vi "Main.vi"() -> ()   [LabVIEW 2017]
doc: "This Continuous Measurement sample project is based on the Queued Message Handler template.\n\nThe Event Handling Loop generates messages based on user interface actions.\n\nThe Message Handling Loop processes messages generated by the Event Handling Loop, or by other messages. There are also Acquisition and Logging message handling loop subVIs, and a chart updating loop."
uses:
  Settings/Settings.ctl
  Acquisition/Hardware Configuration.ctl
  Acquisition/Signal Type.ctl
  Logging/Logging Configuration.ctl
  controls/UI Data.ctl
  controls/UI State.ctl
  support/Message Queue/Enqueue Message (Single).vi
  support/Message Queue/Enqueue Message (Array).vi
  <vilib>/Utility/error.llb/Error Cluster From Error Code.vi
  <vilib>/ErrorRing/Error Ring.xnode
  Acquisition/Acquisition.lvlib
  Logging/Logging.lvlib
  Settings/Settings.lvlib
  support/User Event - Stop/User Event - Stop.lvlib
  support/Message Queue/Message Queue.lvlib
  Settings/Settings Dialog.vi
panel:
  in  "Zero run?":bool
  out "Max writing time to a file [min]":dbl
  out "Elapsed time":timestamp
  out "Test time zero run [s]":dbl
  out "Test time [s]":dbl
  in  "Start":bool
  in  "Stop":bool
  in  "Settings":bool
  out "Status":string
  in  "Exit":bool
  out "Log File Offsite Path":path
  out "Project code":string
  out "Offsite storage?":bool
  out "Log File Path":path
  out "Data":waveform(dbl)[](graph)
  # "Continuous Measurement Data Logger"
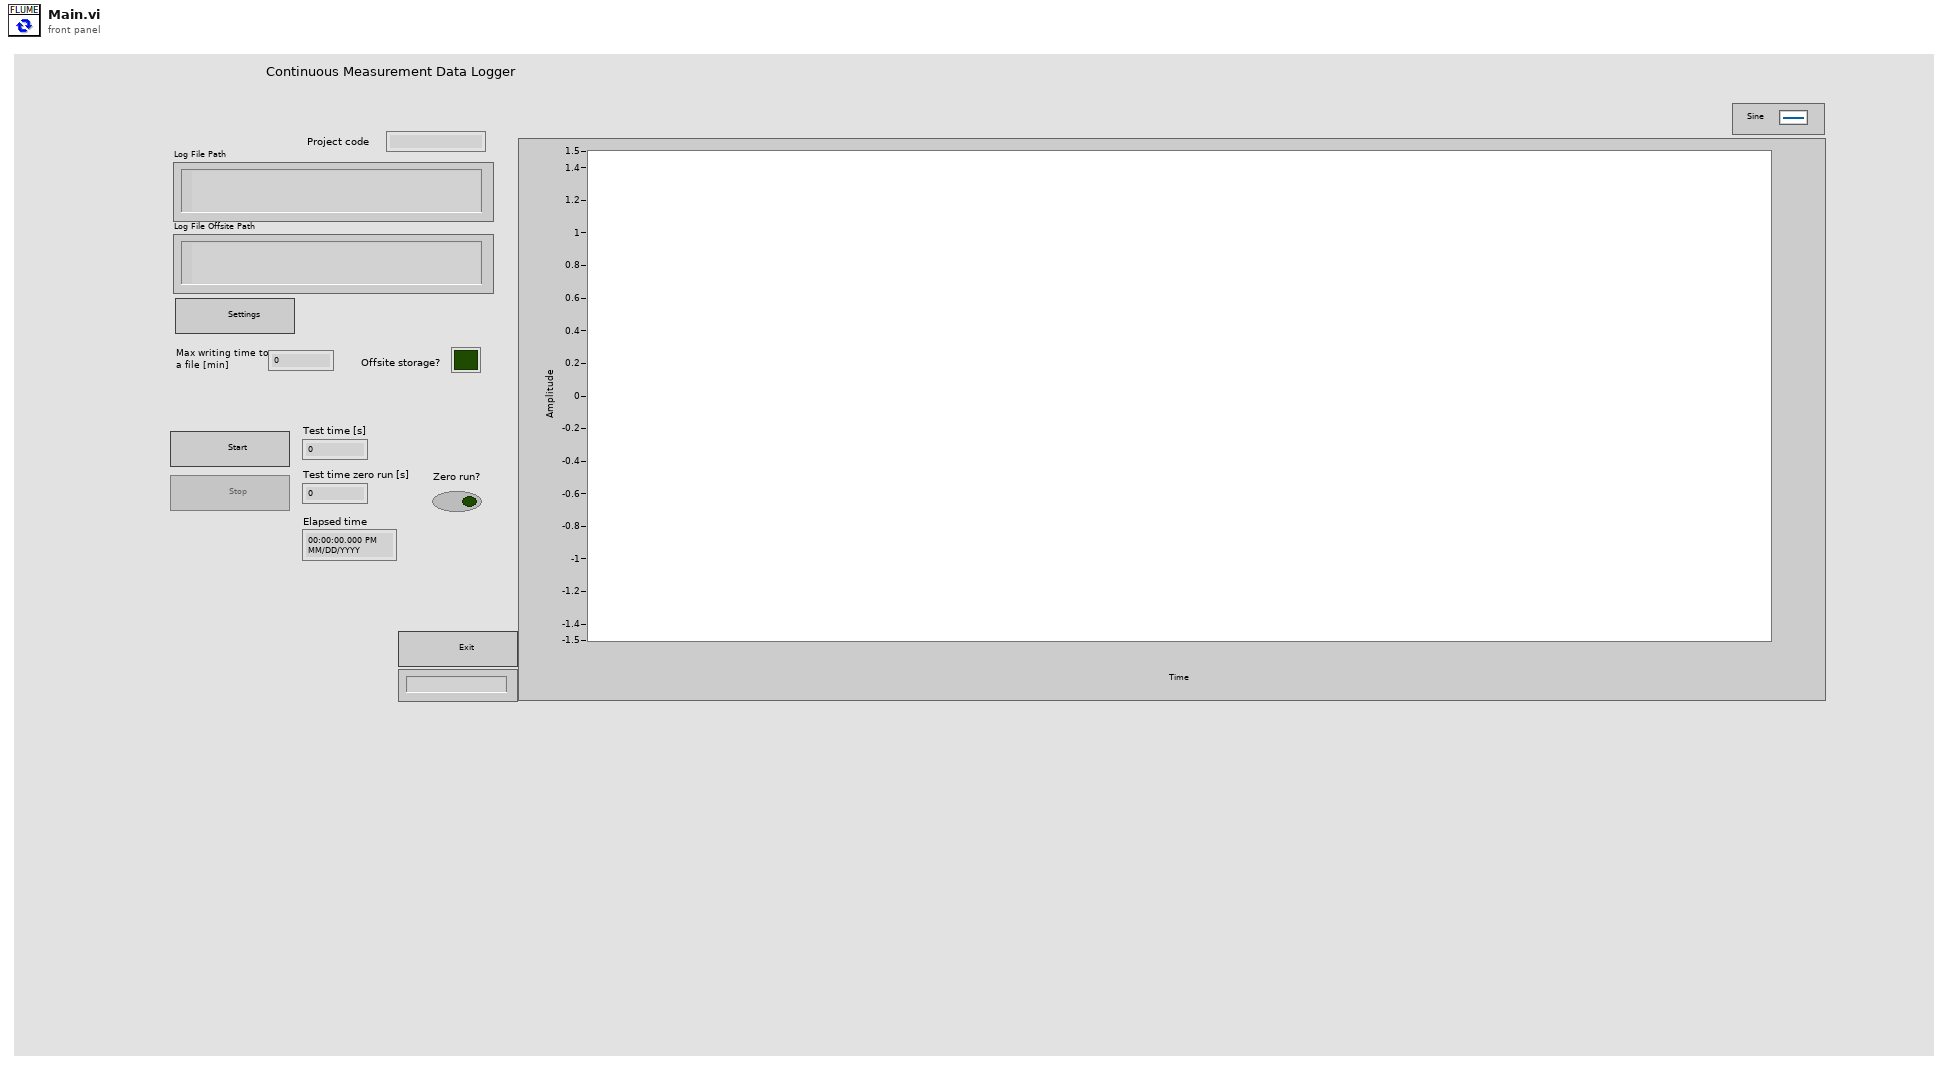
[diagram p1: front panel]
types:
  T1 = typedef "UI State.ctl" = enum16{"Idle", "Acquiring and Logging", "Waiting for Exit", "Waiting for Exit (Acq Stopped)", "Waiting for Exit (Log Stopped)", "Waiting for Stop", "Waiting for Stop (Acq Stopped)", "Waiting for Stop (Log Stopped)"}
  T2 = typedef "UI Data.ctl" = cluster{"Start Ref":refnum<vi>, "Stop Ref":refnum<vi>, "Settings Ref":refnum<vi>, "Exit Ref":refnum<vi>, "Status Ref":refnum<vi>, "Data Ref":refnum<vi>}
  T3 = typedef "Settings.lvlib/Settings.ctl" = cluster{"Hardware Configuration":T4, "Logging Configuration":T6, "Cluster":cluster{"Elapsed Time":dbl, "Test time [s]":dbl, "Test time zero run[s] ":dbl, "Zero run?":bool}}
  T4 = typedef "Acquisition.lvlib/Hardware Configuration.ctl" = cluster{"HW Refnum <Replace Me>":string, "Signal Type <Replace Me>":T5}
  T5 = typedef "Acquisition.lvlib/Signal Type.ctl" = enum16{"Sine Wave", "Square with Noise"}
  T6 = typedef "Logging.lvlib/Logging Configuration.ctl" = cluster{"Log File Base Path":path, "TDMS File Reference":refnum<k34>, "Log File Offsite Path":path, "Offsite storage?":bool, "Project code":string, "Max writing time to a file [min]":dbl}
  T7 = typedef "Message Queue.lvlib/All Message Queues.ctl" = cluster{"UI":refnum<queue>, "Acquisition":refnum<queue>, "Logging":refnum<queue>}
  T8 = cluster{"Elapsed Time":dbl, "Test time [s]":dbl, "Test time zero run[s] ":dbl, "Zero run?":bool}
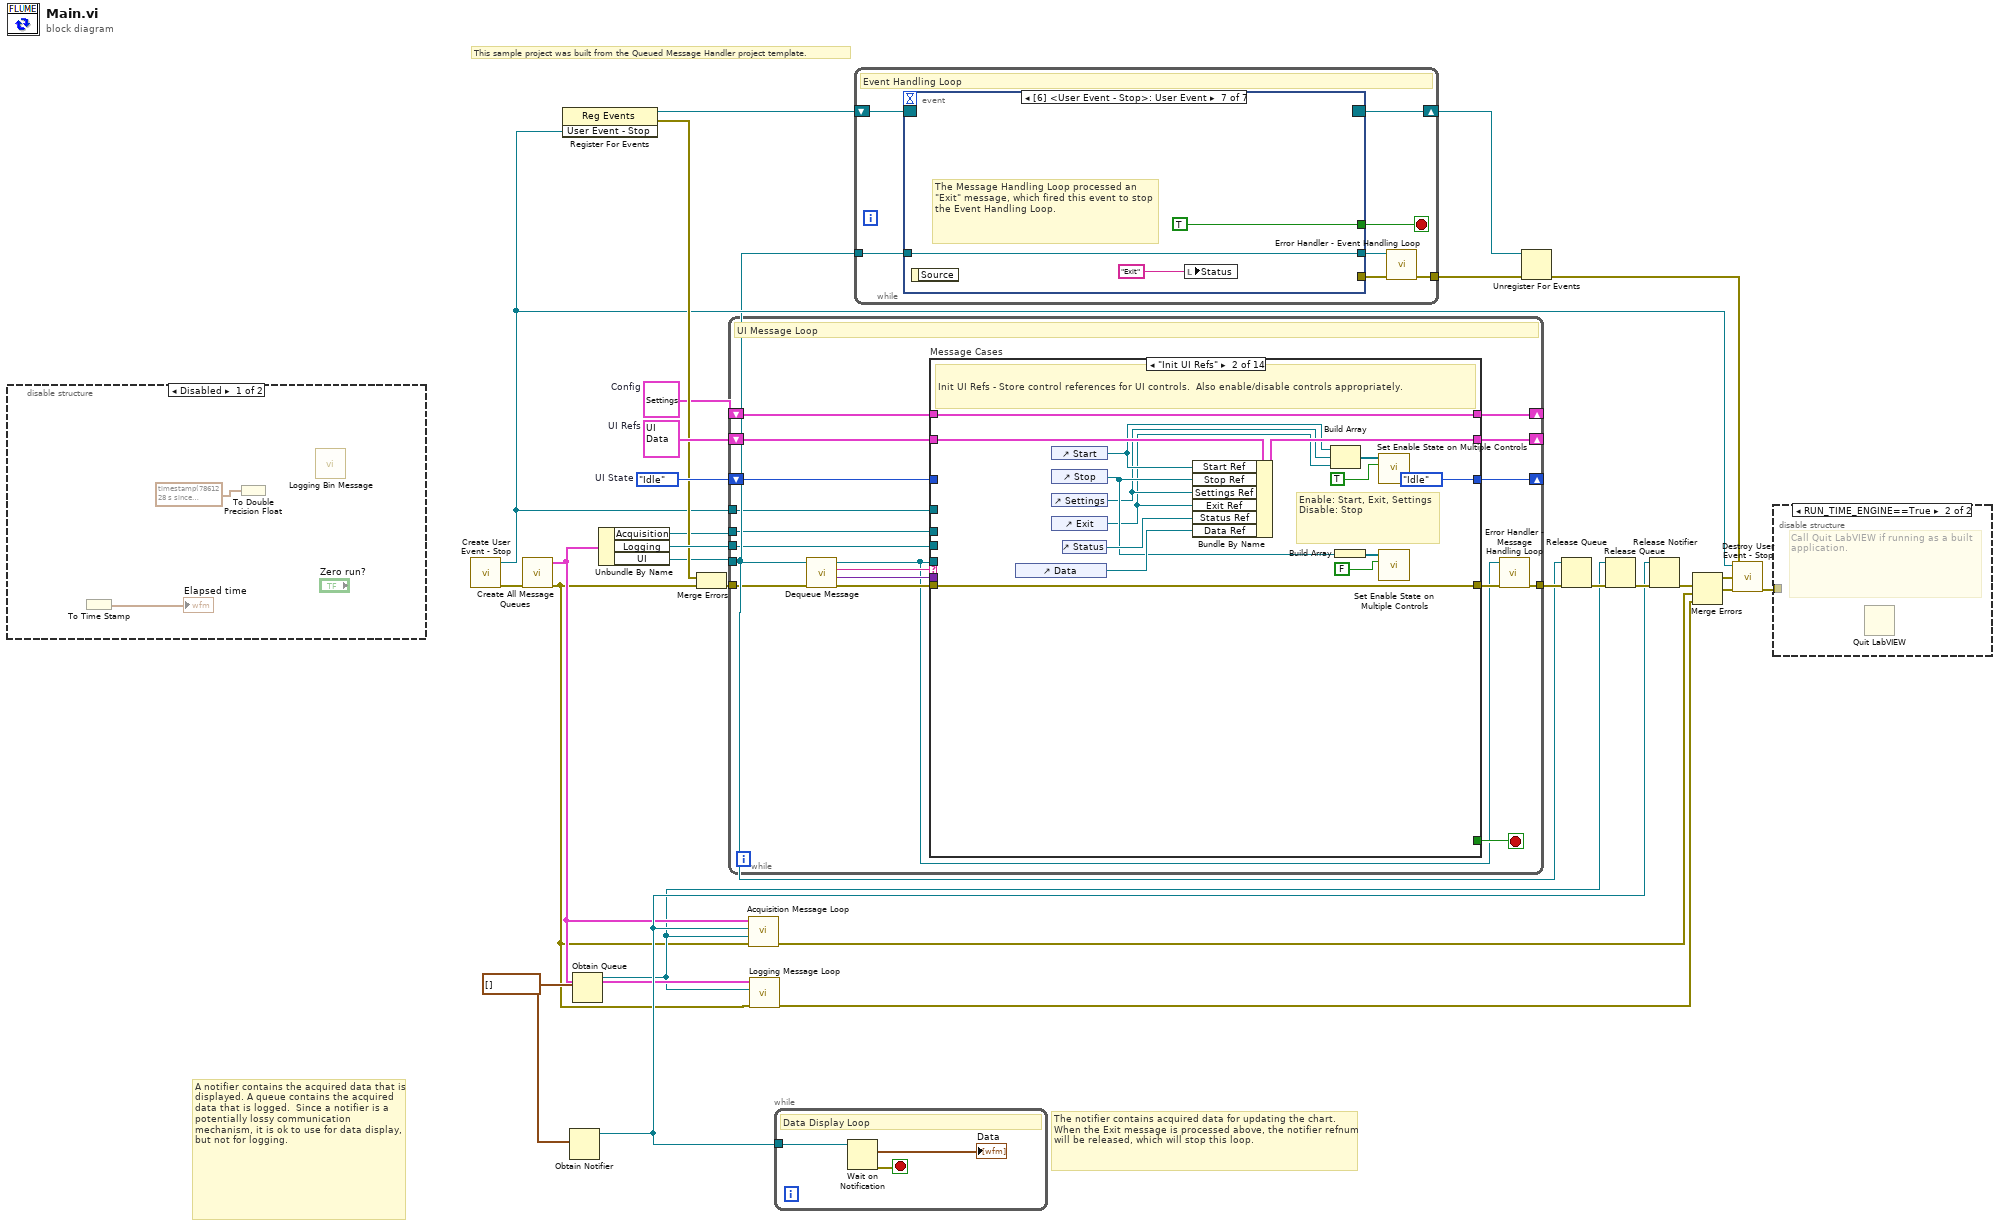
[diagram p0: block diagram]
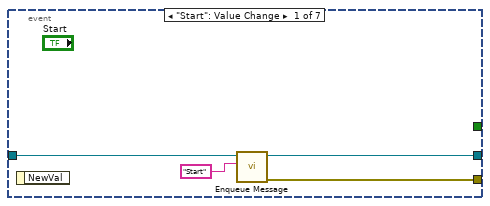
[diagram p4: hidden frame]
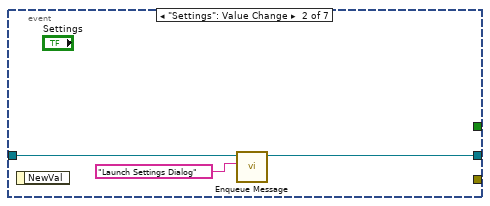
[diagram p5: hidden frame]
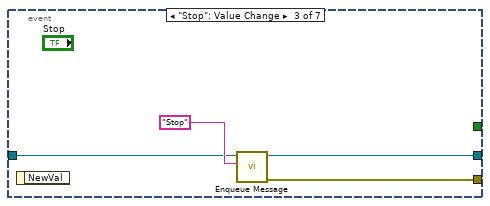
[diagram p6: hidden frame]
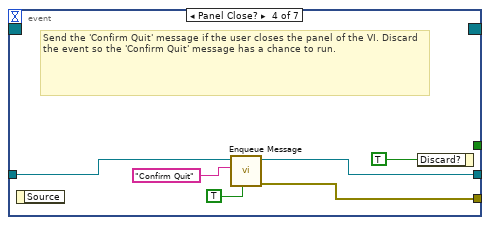
[diagram p7: hidden frame]
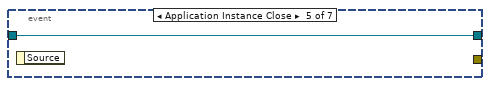
[diagram p8: hidden frame]
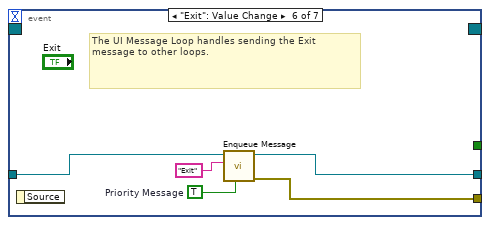
[diagram p9: hidden frame]
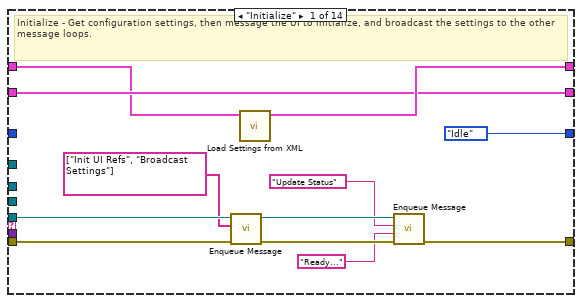
[diagram p10: hidden frame]
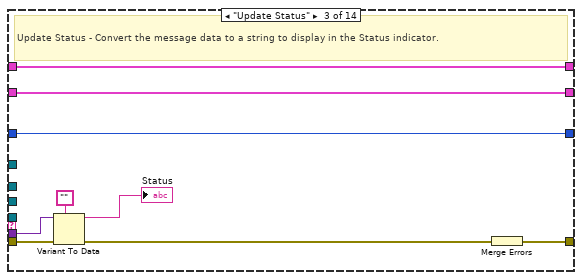
[diagram p11: hidden frame]
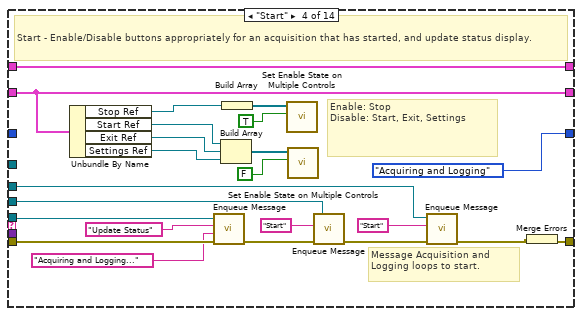
[diagram p12: hidden frame]
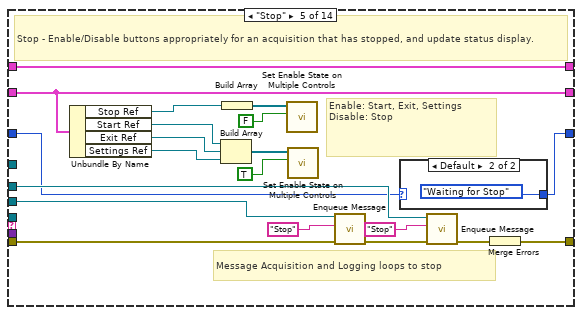
[diagram p13: hidden frame]
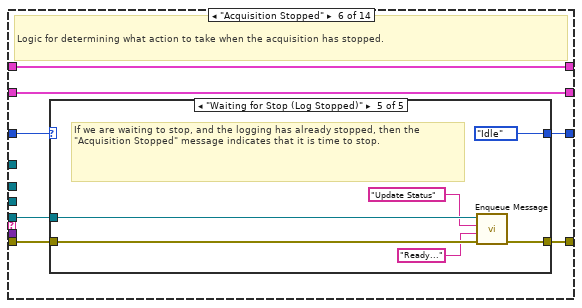
[diagram p15: hidden frame]
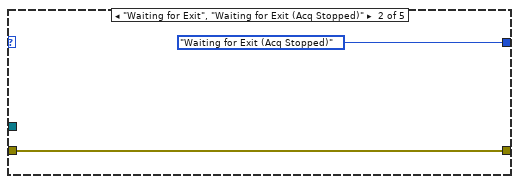
[diagram p17: hidden frame]
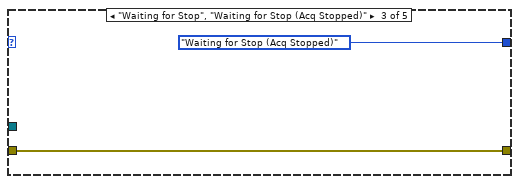
[diagram p18: hidden frame]
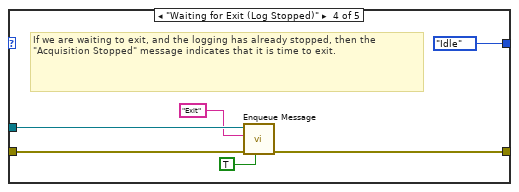
[diagram p19: hidden frame]
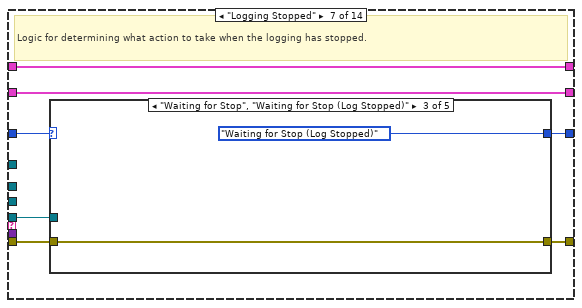
[diagram p20: hidden frame]
diagram:
  w19 = UI_State."Idle"  # UI State
  w4 = waveform(dbl)[] []
  w21 = T2 {"Start Ref"=refnum, "Stop Ref"=refnum, "Settings Ref"=refnum, "Exit Ref"=refnum, "Status Ref"=refnum, "Data Ref"=refnum}  # UI Refs
  w5 = T3 {"Hardware Configuration"={"HW Refnum <Replace Me>"="", "Signal Type <Replace Me>"=enum."Sine Wave"}, "Logging Configuration"={"Log File Base Path"=path "", "TDMS File Reference"=refnum, "Log File Offsite Path"=path "", "Offsite storage?"=FALSE, "Project code"="", "Max writing time to a file [min]"=0.0}, "Cluster"={"Elapsed Time"=0.0, "Test time [s]"=0.0, "Test time zero run[s] "=0.0, "Zero run?"=FALSE}}  # Config
  # "This sample project was built from the Queued Message Handler project template."
  # "A notifier contains the acquired data that is displayed. A queue contains the acquired data that is logged.  Since a notifier is a potentially lossy communication mechanism, it is ok to use for data display, but not for logging."
  # "The notifier contains acquired data for updating the chart. When the Exit message is processed above, the notifier refnum will be released, which will stop this loop."
  n1 = disable-structure shown="Disabled" {
    frame Disabled {
      n2 = To Time Stamp() -> (0:→"Elapsed time":timestamp)  [unwired: 1 in]
      n3 = To Double Precision Float(number=timestamp(7861228 s since 1904-01-01)) -> ()  [unwired: 1 out]
      n4 = call "Logging Bin Message.vi"() -> ()  [unwired: 11 in, 1 out]
    }
    frame Enabled {
    }
  }
  n5 = call "Create User Event - Stop.vi"() -> ("error out"=w24:errorcluster, "User Event - Stop"=w10:refnum<user-event>)  [unwired: 10 in]
  n6 = call "Create All Message Queues.vi"("error in (no error)"=w24) -> ("error out"=w1:errorcluster, "Message Queues out"=w3:T7)  [unwired: 9 in]
  n7 = register-events(w10) -> (reference out=w13:refnum<event-registration>, error out=w11:errorcluster)  [unwired: 2 in]
  n8 = Obtain Notifier(notification data type=w4) -> (notifier out=w6:refnum<notifier>)  [unwired: 3 in, 2 out]
  n9 = Obtain Queue(element data type=w4) -> (queue out=w2:refnum<queue>)  [unwired: 4 in, 2 out]
  n10 = Unbundle By Name(w3) -> ("Acquisition"=w8:refnum<queue>, "Logging"=w20:refnum<queue>, "UI"=w9:refnum<queue>)
  n11 = Merge Errors(w11, w1) -> (w12:errorcluster)
  n12 = while {
    tunnel: w9 -> [w32]
    tunnel: w10 -> [w46]
    shift-right: [w41] -> _
    shift-left: w5 -> [w40]
    shift-right: [w38] -> _
    shift-left: w21 -> [w39]
    tunnel: w8 -> [w37]
    tunnel: w20 -> [w31]
    shift-right: [w33] -> _
    shift-left: w19 -> [w34]
    tunnel: w12 -> [w45]
    tunnel: [w36] -> w27
    stop <- w47 stop-if-true
    # "UI Message Loop"
    n13 = call "Dequeue Message.vi"("error in (no error)"=w45, "Message Queue"=w32) -> ("error out"=w44:errorcluster, "Message Data"=w42:variant, "Message"=w43:string, "dup Message Queue"=w30:refnum<queue>)  [unwired: 6 in]
    n14 = case "Message Cases" shown="\"Init UI Refs\"" w43 {
      selector: w43 -> [_ _ _ _ _ _ _ _ _ _ _ _ _ w272]
      tunnel: w30 -> [w52 _ _ w85 _ w132 w157 _ w204 _ w226 _ _ _]
      tunnel: w44 -> [w51 w74 w82 w106 w125 w133 w158 w193 w206 w214 w225 w254 w270 _]
      tunnel: [w56 w74 w83 w87 w126 w130 w155 w198 w200 w217 w224 w263 w269 w271] -> w35
      tunnel: [_ _ _ _ _ _ _ _ _ _ _ TRUE _ _] -> w47
      tunnel: w42 -> [_ _ w81 _ _ _ _ _ _ w218 _ w252 _ _]
      tunnel: w46 -> [_ _ _ _ _ _ _ _ _ _ _ w264 _ _]
      tunnel: [w59 w60 w75 w84 w107 w129 w154 w196 w199 w213 w222 w250 w268 w275] -> w41
      tunnel: w40 -> [w48 w60 w75 w84 w107 w129 w154 w196 w207 w213 w222 w250 w268 w275]
      tunnel: w39 -> [w53 w73 w77 w103 w124 w135 w160 w191 w202 w221 w228 w262 w267 w274]
      tunnel: [w53 w70 w77 w103 w124 w135 w160 w191 w202 w221 w228 w262 w267 w274] -> w38
      tunnel: w37 -> [_ _ _ w86 w111 _ _ w190 _ _ _ w261 _ _]
      tunnel: w31 -> [_ _ _ w92 w114 _ _ w189 _ _ _ w260 _ _]
      tunnel: w34 -> [_ _ w76 _ w108 w134 w159 w188 w201 w216 w227 _ w266 w273]
      tunnel: [UI_State."Idle" ("UI State") UI_State."Idle" ("UI State") w76 UI_State."Acquiring and Logging" ("UI State") w109 w131 w156 w188 w201 w216 w223 UI_State."Idle" ("UI State") w266 w273] -> w33
      frame "Initialize" {
        # "Initialize - Get configuration settings, then message the UI to initialize, and broadcast the settings to the other message loops."
        n15 = call-poly "Enqueue Message.vi"("error in (no error)"=w51, "Message Array"=string[] ["Init UI Refs", "Broadcast Settings"], "Message Queue"=w52) -> ("error out"=w58:errorcluster, "dup Message Queue"=w57:refnum<queue>)  [unwired: 7 in]
        n16 = call "Load Settings from XML.vi"("Settings in"=w48) -> ("Settings out"=w59:T3)  [unwired: 9 in, 1 out]
        n17 = call-poly "Enqueue Message.vi"("error in (no error)"=w58, "Message Data"="Ready..." ("Ready..."), "Message"="Update Status", "Message Queue"=w57) -> ("error out"=w56:errorcluster)  [unwired: 6 in, 1 out]
      }
      frame "Init UI Refs" {
        # "Enable: Start, Exit, Settings\nDisable: Stop"
        # "Init UI Refs - Store control references for UI controls.  Also enable/disable controls appropriately."
        n18 = control-ref of="Data"() -> (w71:refnum<vi>)
        n19 = control-ref of="Start"() -> (w64:refnum<vi>)
        n20 = control-ref of="Stop"() -> (w65:refnum<vi>)
        n21 = control-ref of="Settings"() -> (w63:refnum<vi>)
        n22 = control-ref of="Exit"() -> (w62:refnum<vi>)
        n23 = control-ref of="Status"() -> (w72:refnum<vi>)
        n24 = Bundle By Name(cluster=w73, "Start Ref"=w64, "Stop Ref"=w65, "Settings Ref"=w63, "Exit Ref"=w62, "Status Ref"=w72, "Data Ref"=w71) -> (w70:T2)
        n25 = Build Array(w64, w63, w62) -> (w68:refnum<vi>[])
        n26 = Build Array(w65) -> (w67:refnum<vi>[])
        n27 = call "Set Enable State on Multiple Controls.vi"("Enable?"=TRUE, "Controls"=w68) -> ()  [unwired: 10 in]
        n28 = call "Set Enable State on Multiple Controls.vi"("Enable?"=FALSE, "Controls"=w67) -> ()  [unwired: 10 in]
      }
      frame "Update Status" {
        # "Update Status - Convert the message data to a string to display in the Status indicator."
        n29 = Variant To Data(error in=w82, type="", Variant=w81) -> (data=→"Status":string, error out=w79:errorcluster)
        n30 = Merge Errors(w79) -> (w83:errorcluster)
      }
      frame "Start" {
        # "Message Acquisition and Logging loops to start."
        # "Enable: Stop\nDisable: Start, Exit, Settings"
        # "Start - Enable/Disable buttons appropriately for an acquisition that has started, and update status display."
        n31 = Unbundle By Name(w103) -> ("Stop Ref"=w98:refnum<vi>, "Start Ref"=w97:refnum<vi>, "Exit Ref"=w96:refnum<vi>, "Settings Ref"=w95:refnum<vi>)
        n32 = call-poly "Enqueue Message.vi"("error in (no error)"=w106, "Message Data"="Acquiring and Logging..." ("Acquiring and Logging..."), "Message"="Update Status", "Message Queue"=w85) -> ("error out"=w94:errorcluster)  [unwired: 6 in, 1 out]
        n33 = Build Array(w97, w96, w95) -> (w101:refnum<vi>[])
        n34 = Build Array(w98) -> (w100:refnum<vi>[])
        n35 = call "Set Enable State on Multiple Controls.vi"("Enable?"=TRUE, "Controls"=w100) -> ()  [unwired: 10 in]
        n36 = call "Set Enable State on Multiple Controls.vi"("Enable?"=FALSE, "Controls"=w101) -> ()  [unwired: 10 in]
        n37 = call-poly "Enqueue Message.vi"("error in (no error)"=w94, "Message"="Start", "Message Queue"=w92) -> ("error out"=w89:errorcluster)  [unwired: 7 in, 1 out]
        n38 = call-poly "Enqueue Message.vi"("error in (no error)"=w89, "Message"="Start", "Message Queue"=w86) -> ("error out"=w88:errorcluster)  [unwired: 7 in, 1 out]
        n39 = Merge Errors(w88) -> (w87:errorcluster)
      }
      frame "Stop" {
        # "Message Acquisition and Logging loops to stop"
        # "Enable: Start, Exit, Settings\nDisable: Stop"
        # "Stop - Enable/Disable buttons appropriately for an acquisition that has stopped, and update status display."
        n40 = Unbundle By Name(w124) -> ("Stop Ref"=w119:refnum<vi>, "Start Ref"=w118:refnum<vi>, "Exit Ref"=w117:refnum<vi>, "Settings Ref"=w116:refnum<vi>)
        n41 = Build Array(w118, w117, w116) -> (w122:refnum<vi>[])
        n42 = Build Array(w119) -> (w121:refnum<vi>[])
        n43 = call "Set Enable State on Multiple Controls.vi"("Enable?"=FALSE, "Controls"=w121) -> ()  [unwired: 10 in]
        n44 = call "Set Enable State on Multiple Controls.vi"("Enable?"=TRUE, "Controls"=w122) -> ()  [unwired: 10 in]
        n45 = call-poly "Enqueue Message.vi"("error in (no error)"=w125, "Message"="Stop", "Message Queue"=w114) -> ("error out"=w113:errorcluster)  [unwired: 7 in, 1 out]
        n46 = case shown="Default" w108 {
          selector: w108 -> [w127 _]
          tunnel: [w127 UI_State."Waiting for Stop" ("UI State")] -> w109
          frame "Waiting for Exit" {
          }
          frame Default {
          }
        }
        n47 = call-poly "Enqueue Message.vi"("error in (no error)"=w113, "Message"="Stop", "Message Queue"=w111) -> ("error out"=w112:errorcluster)  [unwired: 7 in, 1 out]
        n48 = Merge Errors(w112) -> (w126:errorcluster)
      }
      frame "Acquisition Stopped" {
        # "Logic for determining what action to take when the acquisition has stopped."
        n49 = case shown="\"Waiting for Stop (Log Stopped)\"" w134 {
          selector: w134 -> [w137 _ _ _ _]
          tunnel: w133 -> [w136 w139 w141 w147 w153]
          tunnel: w132 -> [_ _ _ w145 w150]
          tunnel: [w137 UI_State."Waiting for Exit (Acq Stopped)" ("UI State") UI_State."Waiting for Stop (Acq Stopped)" ("UI State") UI_State."Idle" ("UI State") UI_State."Idle" ("UI State")] -> w131
          tunnel: [w136 w139 w141 w146 w151] -> w130
          frame Default {
          }
          frame "Waiting for Exit", "Waiting for Exit (Acq Stopped)" {
          }
          frame "Waiting for Stop", "Waiting for Stop (Acq Stopped)" {
          }
          frame "Waiting for Exit (Log Stopped)" {
            # "If we are waiting to exit, and the logging has already stopped, then the \"Acquisition Stopped\" message indicates that it is time to exit."
            n50 = call-poly "Enqueue Message.vi"("Priority Message? (F)"=TRUE, "error in (no error)"=w147, "Message"="Exit", "Message Queue"=w145) -> ("error out"=w146:errorcluster)  [unwired: 6 in, 1 out]
          }
          frame "Waiting for Stop (Log Stopped)" {
            # "If we are waiting to stop, and the logging has already stopped, then the \"Acquisition Stopped\" message indicates that it is time to stop."
            n51 = call-poly "Enqueue Message.vi"("error in (no error)"=w153, "Message Data"="Ready..." ("Ready..."), "Message"="Update Status", "Message Queue"=w150) -> ("error out"=w151:errorcluster)  [unwired: 6 in, 1 out]
          }
        }
      }
      frame "Logging Stopped" {
        # "Logic for determining what action to take when the logging has stopped."
        n52 = case shown="\"Waiting for Stop\", \"Waiting for Stop (Log Stopped)\"" w159 {
          selector: w159 -> [w162 _ _ _ _]
          tunnel: w158 -> [w161 w164 w166 w172 w175]
          tunnel: w157 -> [_ _ _ w170 w174]
          tunnel: [w162 UI_State."Waiting for Exit (Log Stopped)" ("UI State") UI_State."Waiting for Stop (Log Stopped)" ("UI State") UI_State."Idle" ("UI State") UI_State."Idle" ("UI State")] -> w156
          tunnel: [w161 w164 w166 w171 w173] -> w155
          frame Default {
          }
          frame "Waiting for Exit", "Waiting for Exit (Log Stopped)" {
          }
          frame "Waiting for Stop", "Waiting for Stop (Log Stopped)" {
          }
          frame "Waiting for Exit (Acq Stopped)" {
            # "If we are waiting to exit, and the acquisition has already stopped, then the \"Logging Stopped\" message indicates that it is time to exit."
            n53 = call-poly "Enqueue Message.vi"("Priority Message? (F)"=TRUE, "error in (no error)"=w172, "Message"="Exit", "Message Queue"=w170) -> ("error out"=w171:errorcluster)  [unwired: 6 in, 1 out]
          }
          frame "Waiting for Stop (Acq Stopped)" {
            # "If we are waiting to stop, and the acquisition has already stopped, then the \"Logging Stopped\" message indicates that it is time to stop."
            n54 = call-poly "Enqueue Message.vi"("error in (no error)"=w175, "Message Data"="Ready..." ("Ready..."), "Message"="Update Status", "Message Queue"=w174) -> ("error out"=w173:errorcluster)  [unwired: 6 in, 1 out]
          }
        }
      }
      frame "Broadcast settings" {
        w192 = "Update Settings" ("Message")
        # "Broadcast settings - Send the 'Update Settings' message to the Logging and Acquisition message loops."
        n55 = Unbundle By Name(w196) -> ("Hardware Configuration"=w195:T4, "Logging Configuration"=w185:T6, "Cluster"=w183:T8)
        n56 = Unbundle By Name(w183) -> ("Test time [s]"=→"Test time [s]":dbl, "Test time zero run[s]"=→"Test time zero run [s]":dbl)
        n57 = Unbundle By Name(w185) -> ("Log File Base Path"=→"Log File Path":path, "Log File Offsite Path"=→"Log File Offsite Path":path, "Offsite storage?"=→"Offsite storage?":bool, "Project code"=→"Project code":string, "Max writing time to a file [min]"=→"Max writing time to a file [min]":dbl)
        n58 = call-poly "Enqueue Message.vi"("Message Data"=w195, "Message"=w192, "Message Queue"=w190) -> ("error out"=w197:errorcluster)  [unwired: 7 in, 1 out]
        n59 = call-poly "Enqueue Message.vi"("error in (no error)"=w197, "Message Data"=w185, "Message"=w192, "Message Queue"=w189) -> ("error out"=w194:errorcluster)  [unwired: 6 in, 1 out]
        n60 = Merge Errors(w194, w193) -> (w198:errorcluster)
      }
      frame "Launch Settings Dialog" {
        # "Launch Settings Dialog - Launch the Settings Dialog when the user clicks the 'Settings' button."
        n61 = call-by-ref "?"("error in (no error)"=w206, "Settings in"=w207) -> ("error out"=w203:errorcluster, "Cancelled?"=w205:bool, "Settings out"=w199:T3)  [unwired: 8 in, 3 out]
        n62 = case shown="False" w205 {
          tunnel: w204 -> [w211 _]
          tunnel: w203 -> [w210 w212]
          tunnel: [w209 w212] -> w200
          frame False {
            n63 = call-poly "Enqueue Message.vi"("error in (no error)"=w210, "Message"="Broadcast Settings", "Message Queue"=w211) -> ("error out"=w209:errorcluster)  [unwired: 7 in, 1 out]
          }
          frame True {
          }
        }
      }
      frame "Error" {
        # "Error - Display an error dialog. This message is sent by the \"Error Handler\" VIs at the end of other loops in this application."
        n64 = Variant To Data(error in=w214, type=errorcluster {"status"=FALSE, "code"=0, "source"=""} ("error constant"), Variant=w218) -> (data=w215:errorcluster, error out=w219:errorcluster)
        n65 = call <vilib>:"Simple Error Handler.vi"("error in (no error)"=w215) -> ()  [unwired: 4 in, 5 out]
        n66 = Merge Errors(w219) -> (w217:errorcluster)
      }
      frame "Confirm Quit" {
        # "Confirm Quit - Message that can confirm whether or not the user wants to exit the application."
        n67 = case shown="\"Acquiring and Logging\"" w227 {
          tunnel: w226 -> [w234 w238]
          tunnel: w225 -> [w233 w237]
          tunnel: [w232 w236] -> w224
          tunnel: [UI_State."Idle" ("UI State") w235] -> w223
          frame Default {
            # "If 'Confirm Quit' comes in while the system is idle, there is no need for a confirmation message."
            n68 = call-poly "Enqueue Message.vi"("Priority Message? (F)"=TRUE, "error in (no error)"=w233, "Message"="Exit", "Message Queue"=w234) -> ("error out"=w232:errorcluster)  [unwired: 6 in, 1 out]
          }
          frame "Acquiring and Logging" {
            n69 = Two Button Dialog(message="Are you sure you want to quit while the acquisition is running?" ("Confirm Quit Message"), 1:"No" ("No"), 2:"Yes" ("Yes")) -> (T button?=w239:bool)
            n70 = case shown="True" w239 {
              tunnel: w238 -> [_ w248]
              tunnel: w237 -> [w244 w249]
              tunnel: [w244 w247] -> w236
              tunnel: [UI_State."Acquiring and Logging" ("UI State") UI_State."Waiting for Exit" ("UI State")] -> w235
              frame False {
                # "User did not want to quit."
              }
              frame True {
                n71 = call-poly "Enqueue Message.vi"("error in (no error)"=w249, "Message"="Stop", "Message Queue"=w248) -> ("error out"=w247:errorcluster)  [unwired: 7 in, 1 out]
              }
            }
          }
        }
      }
      frame "Exit" {
        w256 = TRUE ("Priority Message? (F)")
        w257 = "Exit" ("Message")
        # "Popup an error dialog if 'Exit' was called as a result of an error."
        # "Stop the VI"
        # "Exit - Send Exit messages to the Acquisition and Logging loops, and fire the user event to stop the Event Handling Loop."
        n72 = Variant To Data(type=errorcluster {"status"=FALSE, "code"=0, "source"=""} ("error constant"), Variant=w252) -> (data=w251:errorcluster)  [unwired: 1 in, 1 out]
        n73 = call <vilib>:"Simple Error Handler.vi"("error in (no error)"=w251) -> ()  [unwired: 4 in, 5 out]
        n74 = call-poly "Enqueue Message.vi"("Priority Message? (F)"=w256, "error in (no error)"=w254, "Message"=w257, "Message Queue"=w261) -> ("error out"=w258:errorcluster)  [unwired: 6 in, 1 out]
        n75 = call-poly "Enqueue Message.vi"("Priority Message? (F)"=w256, "error in (no error)"=w258, "Message"=w257, "Message Queue"=w260) -> ("error out"=w255:errorcluster)  [unwired: 6 in, 1 out]
        n76 = call "Fire User Event - Stop.vi"("error in (no error)"=w255, "User Event - Stop"=w264) -> ("error out"=w263:errorcluster)  [unwired: 9 in]
      }
      frame "---Copy This Frame---" {
        (unwired) FALSE ("Time has Elapsed")
        # "Duplicate this frame when creating new messages.  Change this comment in the duplicated frame to describe this message."
        n77 = Merge Errors(w270) -> (w269:errorcluster)
      }
      frame Default {
        # "'Default' case only runs if there is a message that isn't defined in any of the other cases.  Output a programming error."
        n78 = xnode "Error Ring"("parameter 0"=w272) -> ("error out"=w271:errorcluster)
      }
    }
    n79 = call "Error Handler - Message Handling Loop.vi"("error in (no error)"=w35, "Message Queue"=w30) -> ("dup error in"=w36:errorcluster)  [unwired: 8 in, 1 out]
  }
  n80 = call "Acquisition Message Loop.vi"("error in (no error)"=w1, "Data Queue"=w2, "Data Notifier"=w6, "Message Queues"=w3) -> ("error out"=w25:errorcluster)  [unwired: 7 in]
  n81 = call "Logging Message Loop.vi"("error in (no error)"=w1, "Data Queue"=w2, "Message Queues"=w3) -> ("error out"=w23:errorcluster)  [unwired: 8 in]
  n82 = while "Data Display Loop" {
    tunnel: w6 -> [w285]
    stop <- w284 stop-if-true
    # "Data Display Loop"
    n83 = Wait on Notification(notifier=w285) -> (notification=→"Data":waveform(dbl)[], error out=w284:errorcluster)  [unwired: 3 in, 2 out]
  }
  n84 = while {
    tunnel: w9 -> [w291]
    tunnel: [w288] -> w26
    shift-right: [w290] -> w22
    shift-left: w13 -> [w292]
    stop <- w289 stop-if-true
    # "Event Handling Loop"
    n85 = event shown="[6] <User Event - Stop>: User Event" {
      selector: w292 -> [_ _ _ _ _ _ _]
      dyn-events: [_ _ _ _ _ _ _] -> w290
      timeout: _ -> [_ _ _ _ _ _ _]
      tunnel: [_ _ _ _ _ _ TRUE ("Discard?")] -> w289
      tunnel: w291 -> [w296 w298 w302 w307 w310 w312 w316]
      tunnel: [w294 _ w301 w305 _ w315 _] -> w287
      tunnel: [w293 w297 w300 w306 w310 w311 w316] -> w286
      event "Start": Value Change {
        n86 = event-data() -> ()  [unwired: 1 in, 1 out]
        n87 = call-poly "Enqueue Message.vi"("Message"="Start", "Message Queue"=w296) -> ("error out"=w294:errorcluster, "dup Message Queue"=w293:refnum<queue>)  [unwired: 8 in]
      }
      event "Settings": Value Change {
        n88 = event-data() -> ()  [unwired: 1 in, 1 out]
        n89 = call-poly "Enqueue Message.vi"("Message"="Launch Settings Dialog", "Message Queue"=w298) -> ("dup Message Queue"=w297:refnum<queue>)  [unwired: 8 in, 1 out]
      }
      event "Stop": Value Change {
        n90 = event-data() -> ()  [unwired: 1 in, 1 out]
        n91 = call-poly "Enqueue Message.vi"("Message"="Stop", "Message Queue"=w302) -> ("error out"=w301:errorcluster, "dup Message Queue"=w300:refnum<queue>)  [unwired: 8 in]
      }
      event Panel Close? {
        # "Send the 'Confirm Quit' message if the user closes the panel of the VI. Discard the event so the 'Confirm Quit' message has a chance to run."
        n92 = event-data() -> ()  [unwired: 1 in, 1 out]
        n93 = call-poly "Enqueue Message.vi"("Priority Message? (F)"=TRUE, "Message"="Confirm Quit", "Message Queue"=w307) -> ("error out"=w305:errorcluster, "dup Message Queue"=w306:refnum<queue>)  [unwired: 7 in]
        n94 = event-data("Discard?"=TRUE) -> ()  [unwired: 1 in, 1 out]
      }
      event Application Instance Close {
        n95 = event-data() -> ()  [unwired: 1 in, 1 out]
      }
      event "Exit": Value Change {
        w313 = TRUE  # Priority Message
        # "The UI Message Loop handles sending the Exit message to other loops."
        n96 = event-data() -> ()  [unwired: 1 in, 1 out]
        n97 = call-poly "Enqueue Message.vi"("Priority Message? (F)"=w313, "Message"="Exit", "Message Queue"=w312) -> ("error out"=w315:errorcluster, "dup Message Queue"=w311:refnum<queue>)  [unwired: 7 in]
      }
      event User Event {
        # "The Message Handling Loop processed an \"Exit\" message, which fired this event to stop the Event Handling Loop."
        n98 = event-data() -> ()  [unwired: 1 in, 1 out]
        n99 = local write "Status"("Exit" ("Exit String")) -> ()
      }
    }
    n100 = call "Error Handler - Event Handling Loop.vi"("error in (no error)"=w287, "Message Queue"=w286) -> ("dup error in"=w288:errorcluster)  [unwired: 8 in, 1 out]
  }
  n101 = Unregister For Events(event registration refnum=w22, error in=w26) -> (error out=w7:errorcluster)
  n102 = Release Queue(queue=w9, error in (no error)=w27) -> (error out=w16:errorcluster)  [unwired: 1 in, 2 out]
  n103 = Release Queue(queue=w2, error in (no error)=w16) -> (error out=w15:errorcluster)  [unwired: 1 in, 2 out]
  n104 = Release Notifier(notifier=w6, error in (no error)=w15) -> (error out=w14:errorcluster)  [unwired: 1 in, 2 out]
  n105 = Merge Errors(w7, w14, w25, w23) -> (w18:errorcluster)
  n106 = call "Destroy User Event - Stop.vi"("error in (no error)"=w18, "User Event - Stop"=w10) -> ("error out"=w17:errorcluster)  [unwired: 9 in]
  n107 = disable-structure shown="RUN_TIME_ENGINE==True" {
    disable-tunnel: w17 -> [_ _]
    frame condition #0 (active) {
    }
    frame condition #1 {
      # "Call Quit LabVIEW if running as a built application."
      n108 = Quit LabVIEW() -> ()  [unwired: 1 in]
    }
  }
